vi "AnalogIntegratorFastOszi_NI5771.vi"() -> ()   [LabVIEW 2012]
uses:
  <vilib>/Platform/TimedLoop/XDataNode/timing_clust.ctl
  <vilib>/Platform/TimedLoop/XDataNode/nitl_modes.ctl
  <vilib>/Platform/TimedLoop/XDataNode/wakeup.ctl
  <vilib>/rvi/FIFO/Fifo_Resource/nirvififoEmulationSetSize.vi
  <vilib>/rvi/DataTransferAndStorage/Container/Common/niFpgaContainerGetUniqueNameForEmu.vi
  <vilib>/rvi/eio/common/nirviEmuTemplateMethod_errors.vi
  <vilib>/rvi/Emulation/niFpgaSctlEmulationRegisterWithScheduler.vi
  <vilib>/rvi/errors/niFpgaSetErrorForExecOnDevCompSimple.vi
  <vilib>/rvi/eio/common/nirviEmuReportErrorAndStop.vi
  <vilib>/rvi/Emulation/niFpgaSctlEmulationFifoFullMgr.vi
  <vilib>/rvi/Emulation/niFpgaSctlEmulationResourceMgr.vi
  <vilib>/rvi/Emulation/niFpgaSctlEmulationScheduler.vi
  <vilib>/rvi/interface/RandomDataEmulation/nirviRandomDataFPGAFIFO.vi
  <vilib>/rvi/interface/RandomDataEmulation/niFpgaRandomDataHandleErrors.vi
  <vilib>/Platform/TimedLoop/XDataNode/XDataNode.xnode
  <vilib>/rvi/DataTransferAndStorage/Container/XNode/niFpgaContainer.xnode
  <vilib>/rvi/FIFO/Fifo_Resource/nirvififoEmulationClear.vi
  <vilib>/eio/EIONode/EIONode.xnode
  <vilib>/rvi/FIFO/Fifo_Resource/nirvififoEmulationWrite.vi
  <vilib>/rvi/FIFO/Fifo_Resource/nirvififoEmulationRead.vi
  <vilib>/rvi/interface/RandomDataEmulation/nirviRandomDataFpgaReadWriteTemplate.vi
  <vilib>/Platform/TimedLoop/XDataNode/XDNodeRunTimeDep.lvlib
panel:
  in  "Baseline U8":u8
  in  "Acquire continuously":bool
  in  "Clear Interloop FIFO":bool
  out "InterloopFIFO Timeout":bool
  out "ToHostCh1FIFO Overflow":bool
  in  "Acquire":bool
  out "InterloopFIFO Overflow":bool
  out "Acquiring":bool
  out "IO Module\\AI Over Range":bool
  in  "Samples to acquire":u32=10000 caption="Samples per pixel Acq"
  in  "User Command Commit":bool
  in  "User Command":u8
  out "User Command Idle":bool
  out "User Command Status":u8
  in  "User Data 0":u16
  in  "User Data 1":u8
  out "PLL Locked":bool
  out "User Error":bool
  out "Configured?":bool
  # "5771 IO module configuration"
  # "Analog integrator Fast Oszi mode"
  # "Acquisition control"
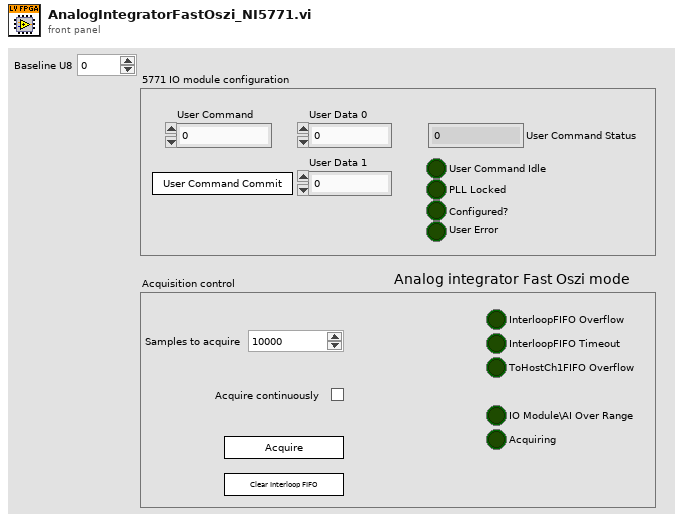
[diagram p1: front panel]
types:
  T1 = typedef "XDNodeRunTimeDep.lvlib/timing_clust.ctl" = cluster{"Expected End [f-1]":u64, "Actual End [f-1]":u64, "Finished Late? [f-1]":bool, "Expected End [i-1]":u64, "Actual End [i-1]":u64, "Finished Late? [i-1]":bool, "Expected Start [i]":u64, "Actual Start [i]":u64, "Expected Start [f]":u64, "Actual Start [f]":u64, "Source Name":string, "Structure Name":string, "Period":i64, "Deadline":i64, "Offset":i64, "Start":i64, "Priority":i32, "Timeout":i32, "Mode":T2, "Wakeup Reason":T3, "Error":errorcluster, "Source Type":string, "Secondary Source Type":string, "Global End Time":u64, "Global Start Time":u64, "Frame Duration":u64, "Iteration Duration":u64, "Assigned CPU":i32, "I/O Scan Engine Mode":u32}
  T2 = typedef "XDNodeRunTimeDep.lvlib/nitl_modes.ctl" = enum32{"No Change", "Process missed periods, maintain original phase", "Discard missed periods, maintain original phase", "Process missed periods, ignore original phase", "Discard missed periods, ignore original phase"}
  T3 = typedef "XDNodeRunTimeDep.lvlib/wakeup.ctl" = enum32{"Normal", "Aborted", "Asynchronous wakeup", "Timing source error", "Timed loop error", "Timeout"}
  T4 = cluster{u64, "IO Module\\Synchronous Trigger Input":u8}
  T5 = cluster{"Data U64":u64, "IO Module\\Synchronous Trigger Input":u8}
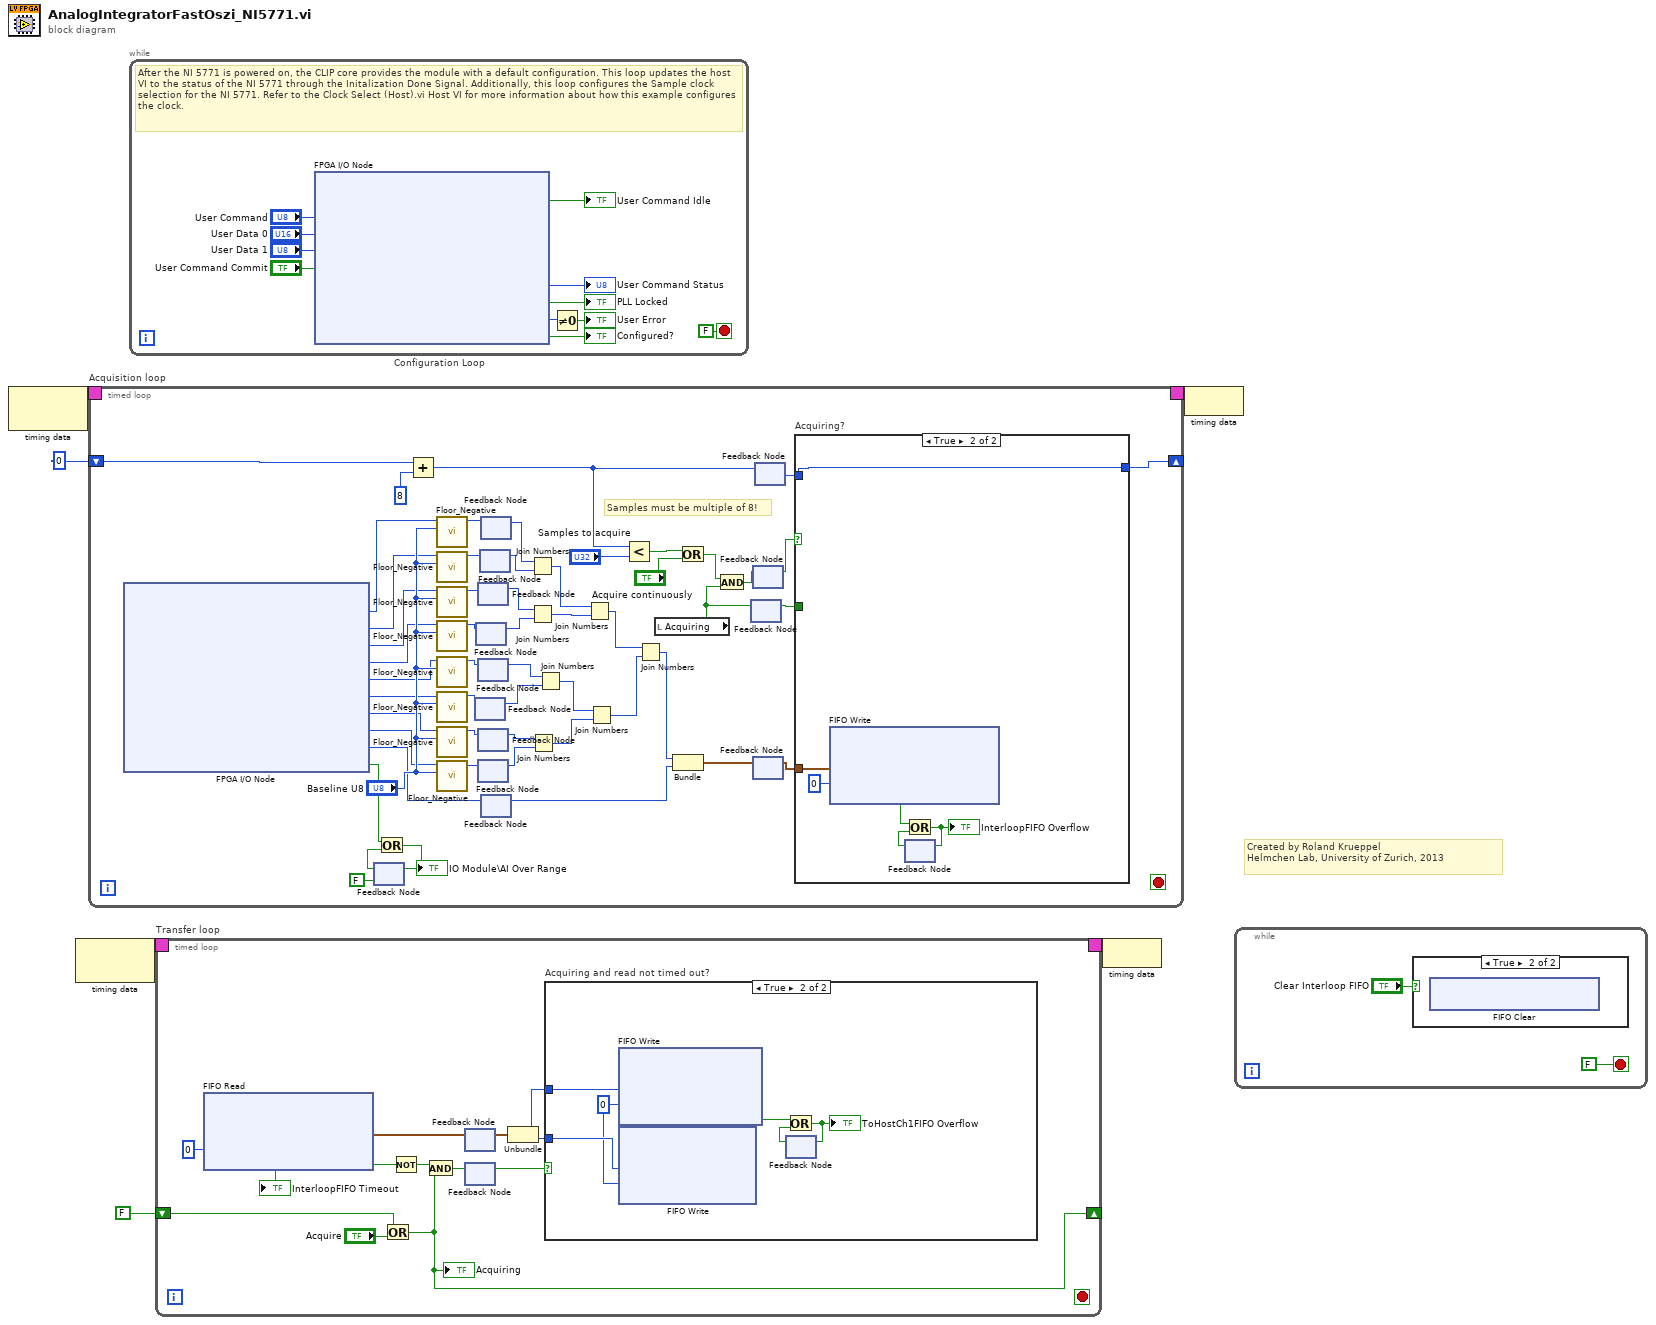
[diagram p0: block diagram]
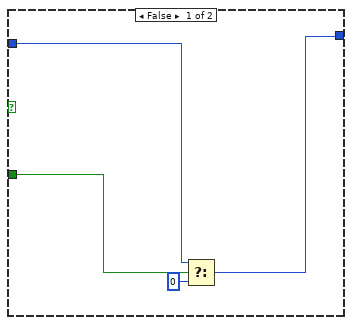
[diagram p4: hidden frame]
diagram:
  # "Created by Roland Krueppel\nHelmchen Lab, University of Zurich, 2013"
  n1 = node-c288() -> (w6:T1)  [unwired: 1 in]
  n2 = node-c288() -> (w3:T1)  [unwired: 1 in]
  n3 = timed-loop "Acquisition loop" {
    timing: w6 -> [_]
    timing-out: [_] -> w5
    shift-right: [w55] -> _
    shift-left: u32 0 ("t") -> [w52]
    stop <- _ stop-if-true
    # "Samples must be multiple of 8!"
    n4 = xnode "FPGA I/O Node"() -> ("IO Module\\AI 0 Data N-7"=w32:u8, "IO Module\\AI 0 Data N-6"=w31:u8, "IO Module\\AI 0 Data N-5"=w30:u8, "IO Module\\AI 0 Data N-4"=w29:u8, "IO Module\\AI 0 Data N-3"=w28:u8, "IO Module\\AI 0 Data N-2"=w25:u8, "IO Module\\AI 0 Data N-1"=w26:u8, "IO Module\\AI 0 Data N"=w27:u8, "IO Module\\Synchronous Trigger Input"=w24:u8, "IO Module\\AI Over Range"=w59:bool)  [unwired: 10 in, 10 out]
    n5 = feedback #1(FALSE) -> (w58:bool)
    n6 = Or(x=w59, y=w58) -> (x .or. y?=w57:bool)
    "IO Module\\AI Over Range" <- w57
    n7 = feedback-in #1(w57) -> ()
    n8 = Add(x=w52, y=u32 8) -> (x+y=w42:u32)
    n9 = call "Floor_Negative.vi"("Baseline U8"="Baseline U8", "Input Value"=w32) -> ("Output Value"=w22:u8)  [unwired: 9 in]
    n10 = call "Floor_Negative.vi"("Baseline U8"="Baseline U8", "Input Value"=w31) -> ("Output Value"=w20:u8)  [unwired: 9 in]
    n11 = call "Floor_Negative.vi"("Baseline U8"="Baseline U8", "Input Value"=w30) -> ("Output Value"=w19:u8)  [unwired: 9 in]
    n12 = call "Floor_Negative.vi"("Baseline U8"="Baseline U8", "Input Value"=w29) -> ("Output Value"=w18:u8)  [unwired: 9 in]
    n13 = call "Floor_Negative.vi"("Baseline U8"="Baseline U8", "Input Value"=w28) -> ("Output Value"=w17:u8)  [unwired: 9 in]
    n14 = call "Floor_Negative.vi"("Baseline U8"="Baseline U8", "Input Value"=w25) -> ("Output Value"=w16:u8)  [unwired: 9 in]
    n15 = call "Floor_Negative.vi"("Baseline U8"="Baseline U8", "Input Value"=w26) -> ("Output Value"=w15:u8)  [unwired: 9 in]
    n16 = call "Floor_Negative.vi"("Baseline U8"="Baseline U8", "Input Value"=w27) -> ("Output Value"=w14:u8)  [unwired: 9 in]
    n17 = feedback #2() -> (w11:u8)  [unwired: 1 in]
    n18 = feedback-in #2(w16) -> ()
    n19 = feedback #3() -> (w9:u8)  [unwired: 1 in]
    n20 = feedback-in #3(w18) -> ()
    n21 = feedback #4() -> (w8:u8)  [unwired: 1 in]
    n22 = feedback-in #4(w19) -> ()
    n23 = feedback #5() -> (w10:u8)  [unwired: 1 in]
    n24 = feedback-in #5(w17) -> ()
    n25 = feedback #6() -> (w12:u8)  [unwired: 1 in]
    n26 = feedback-in #6(w15) -> ()
    n27 = feedback #7() -> (w13:u8)  [unwired: 1 in]
    n28 = feedback-in #7(w14) -> ()
    n29 = feedback #8() -> (w7:u8)  [unwired: 1 in]
    n30 = feedback-in #8(w20) -> ()
    n31 = feedback #9() -> (w21:u8)  [unwired: 1 in]
    n32 = feedback-in #9(w22) -> ()
    n33 = feedback #10() -> (w23:u8)  [unwired: 1 in]
    n34 = feedback-in #10(w24) -> ()
    n35 = Join Numbers(hi=w21, lo=w7) -> ((hi.lo)=w51:u16)
    n36 = Join Numbers(hi=w8, lo=w9) -> ((hi.lo)=w50:u16)
    n37 = Join Numbers(hi=w12, lo=w13) -> ((hi.lo)=w48:u16)
    n38 = Join Numbers(hi=w10, lo=w11) -> ((hi.lo)=w49:u16)
    n39 = Join Numbers(hi=w51, lo=w50) -> ((hi.lo)=w47:u32)
    n40 = Join Numbers(hi=w49, lo=w48) -> ((hi.lo)=w46:u32)
    n41 = Less?(x=w42, y="Samples to acquire") -> (x < y?=w36:bool)
    n42 = Join Numbers(hi=w47, lo=w46) -> ((hi.lo)=w45:u64)
    n43 = local read "Acquiring"() -> (w38:bool)
    n44 = Bundle(w45, "IO Module\\Synchronous Trigger Input"=w23) -> (w44:T4)  [unwired: 1 in]
    n45 = Or(x=w36, y="Acquire continuously") -> (x .or. y?=w34:bool)
    n46 = And(x=w34, y=w38) -> (x .and. y?=w40:bool)
    n47 = feedback #11() -> (w37:bool)  [unwired: 1 in]
    n48 = feedback-in #11(w38) -> ()
    n49 = feedback #12() -> (w39:bool)  [unwired: 1 in]
    n50 = feedback-in #12(w40) -> ()
    n51 = feedback #13() -> (w43:T4)  [unwired: 1 in]
    n52 = feedback-in #13(w44) -> ()
    n53 = feedback #14() -> (w41:u32)  [unwired: 1 in]
    n54 = feedback-in #14(w42) -> ()
    n55 = case "Acquiring?" shown="True" w39 {
      tunnel: [w60 w64] -> w55
      tunnel: w43 -> [_ w69]
      tunnel: w41 -> [w62 w64]
      tunnel: w37 -> [w63 _]
      frame False {
        n56 = Select(t=w62, s=w63, f=u16 0 ("t")) -> (s? t:f=w60:u32)
      }
      frame True {
        n57 = xnode ("FIFO Write")("Element"=w69, "Timeout"=0) -> ("Timed Out?"=w67:bool)  [unwired: 1 in, 1 out]
        n58 = feedback #15() -> (w65:bool)  [unwired: 1 in]
        n59 = Or(x=w67, y=w65) -> (x .or. y?=w66:bool)
        "InterloopFIFO Overflow" <- w66
        n60 = feedback-in #15(w66) -> ()
      }
    }
  }
  n61 = while "Configuration Loop" {
    stop <- FALSE stop-if-true
    # "After the NI 5771 is powered on, the CLIP core provides the module with a default configuration. This loop updates the host VI to the status of the NI 5771 through the Initalization Done Signal. Additionally, this loop configures the Sample clock selection for the NI 5771. Refer to the Clock Select (Host).vi Host VI for more information about how this example configures the clock."
    n62 = xnode "FPGA I/O Node"("IO Module\\User Command"="User Command", "IO Module\\User Data 0"="User Data 0", "IO Module\\User Data 1"="User Data 1", "IO Module\\User Command Commit"="User Command Commit") -> ("IO Module\\User Command Idle"=→"User Command Idle":bool, "IO Module\\User Command Status"=→"User Command Status":u8, "IO Module\\PLL Locked"=→"PLL Locked":bool, "IO Module\\User Error"=w75:u8, "IO Module\\Initialization Done"=→"Configured?":bool)  [unwired: 9 in, 9 out]
    n63 = Not Equal To 0?(x=w75) -> (x != 0?=→"User Error":bool)
  }
  n64 = timed-loop "Transfer loop" {
    timing: w3 -> [_]
    timing-out: [_] -> w2
    shift-right: [w91] -> _
    shift-left: FALSE -> [w89]
    stop <- _ stop-if-true
    n65 = xnode ("FIFO Read")("Timeout"=0) -> ("Element"=w86:T5, "Timed Out?"=w93:bool)  [unwired: 1 in, 1 out]
    "InterloopFIFO Timeout" <- w93
    n66 = Or(x=w89, y="Acquire") -> (x .or. y?=w91:bool)
    "Acquiring" <- w91
    n67 = Not(x=w93) -> (.not. x?=w92:bool)
    n68 = And(x=w92, y=w91) -> (x .and. y?=w84:bool)
    n69 = feedback-in #16(w86) -> ()
    n70 = feedback #16() -> (w85:T5)  [unwired: 1 in]
    n71 = feedback #17() -> (w83:bool)  [unwired: 1 in]
    n72 = feedback-in #17(w84) -> ()
    n73 = Unbundle(w85) -> ("Data U64"=w88:u64, "IO Module\\Synchronous Trigger Input"=w87:u8)
    n74 = case "Acquiring and read not timed out?" shown="True" w83 {
      tunnel: w88 -> [_ w97]
      tunnel: w87 -> [_ w96]
      frame False {
      }
      frame True {
        w95 = 0 ("Timeout")
        n75 = xnode ("FIFO Write")("Element"=w97, "Timeout"=w95) -> ("Timed Out?"=w99:bool)  [unwired: 1 in, 1 out]
        n76 = xnode ("FIFO Write")("Element"=w96, "Timeout"=w95) -> ()  [unwired: 1 in, 2 out]
        n77 = feedback #18() -> (w98:bool)  [unwired: 1 in]
        n78 = Or(x=w99, y=w98) -> (x .or. y?=w100:bool)
        "ToHostCh1FIFO Overflow" <- w100
        n79 = feedback-in #18(w100) -> ()
      }
    }
  }
  n80 = node-c288(w2) -> ()
  n81 = node-c288(w5) -> ()
  n82 = while {
    stop <- FALSE stop-if-true
    n83 = case shown="True" "Clear Interloop FIFO" {
      frame False {
      }
      frame True {
        n84 = xnode ("FIFO Clear")() -> ()  [unwired: 1 in, 1 out]
      }
    }
  }
